vi "RunJustTailEllipseRatioRails.vi"() -> ()   [LabVIEW 2019]
uses:
  Parameters.ctl
  JustTailEllipseRatioRails/JustTailEllipseRatioRailsInputCluster.ctl
  JustTailEllipseRatioRails.lvclass
  D:/Github_repos/ProjectAPI/LabviewVIs/StimulusObject.lvclass
panel:
  in  "JustTailEllipseRatioRailsInputCluster":T1={"Constant Intensity (uW/mm^2, negative is blue)"=0.0, "dot radius (mm)"=0.2, "Intensities (uW/mm^2, negative is blue)"=[], "Durations (s)"=[], "Inter trigger interval (s)"=30.0, "Ellipse Ratio Trigger Point"=5.0}
  out "error IO":errorcluster
  in  "SSH password 2":string
  in  "SSH user name 2":string
  in  "Start":bool
  in  "Wait Before Recording (s)":u32
  in  "SSH password":string
  in  "SSH user name":string
  in  "Last Experiment of the Day":bool
  in  "Tags":string
  out "Parameters":T2 {"FW_WormLengthSD" format="%#.6e"}
  # "Faux Worm Drawing"
  # "Tracking"
  # "Temporal Calibration"
  # "Stimulus Generation"
  # "Median Filtering"
  # "Experimental Settings"
  # "Camera and Projector Settings"
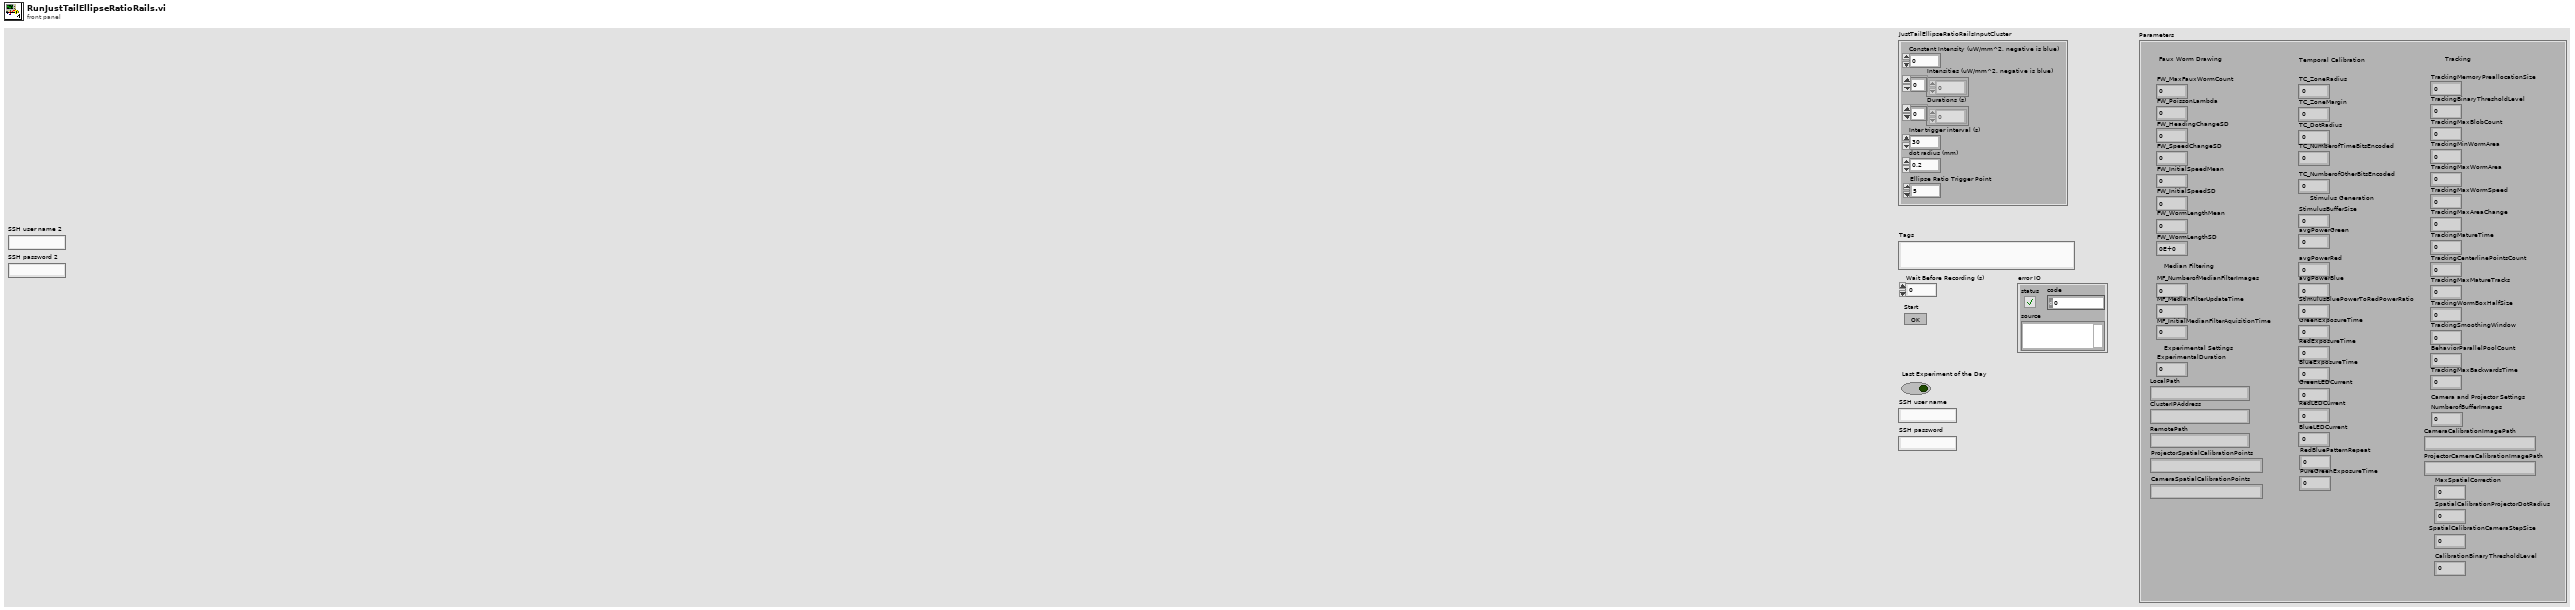
[diagram p1: front panel]
types:
  T1 = typedef "JustTailEllipseRatioRails.lvclass/JustTailEllipseRatioRailsInputCluster.ctl" = cluster{"Constant Intensity (uW/mm^2, negative is blue)":sgl, "dot radius (mm)":sgl, "Intensities (uW/mm^2, negative is blue)":sgl[], "Durations (s)":sgl[], "Inter trigger interval (s)":dbl, "Ellipse Ratio Trigger Point":sgl}
  T2 = typedef "Parameters.ctl" = cluster{"FW_MaxFauxWormCount":i32, "FW_PoissonLambda":dbl, "FW_HeadingChangeSD":dbl, "FW_SpeedChangeSD":dbl, "FW_InitialSpeedMean":dbl, "FW_InitialSpeedSD":dbl, "FW_WormLengthMean":dbl, "FW_WormLengthSD":dbl, "MF_NumberofMedianFilterImages":i32, "MF_MedianFilterUpdateTime":i32, "MF_InitialMedianFilterAquisitionTime":dbl, "ExperimentalDuration":i32, "TC_ZoneRadius":i32, "TC_ZoneMargin":i32, "TC_DotRadius":dbl, "TC_NumberofTimeBitsEncoded":i32, "TC_NumberofOtherBitsEncoded":i32, "NumberofBufferImages":sgl, "CameraCalibrationImagePath":string, "ProjectorCameraCalibrationImagePath":string, "StimulusBufferSize":i32, "TrackingMemoryPreallocationSize":i32, "TrackingBinaryThresholdLevel":sgl, "TrackingMaxBlobCount":i32, "TrackingMinWormArea":dbl, "TrackingMaxWormArea":dbl, "TrackingMaxWormSpeed":dbl, "TrackingMaxAreaChange":dbl, "TrackingMatureTime":i32, "TrackingCenterlinePointsCount":i32, "TrackingMaxMatureTracks":i32, "TrackingWormBoxHalfSize":i32, "TrackingSmoothingWindow":i32, "BehaviorParallelPoolCount":i32, "LocalPath":string, "GreenExposureTime":i32, "RedExposureTime":i32, "BlueExposureTime":i32, "ClusterIPAddress":string, "RemotePath":string, "GreenLEDCurrent":u8, "RedLEDCurrent":u8, "BlueLEDCurrent":u8, "avgPowerGreen":sgl, "avgPowerRed":sgl, "avgPowerBlue":sgl, "StimulusBluePowerToRedPowerRatio":sgl, "TrackingMaxBackwardsTime":i32, "MaxSpatialCorrection":dbl, "ProjectorSpatialCalibrationPoints":string, "SpatialCalibrationProjectorDotRadius":i32, "SpatialCalibrationCameraStepSize":dbl, "CameraSpatialCalibrationPoints":string, "CalibrationBinaryThresholdLevel":dbl, "RedBluePatternRepeat":i32, "PureGreenExposureTime":i32}
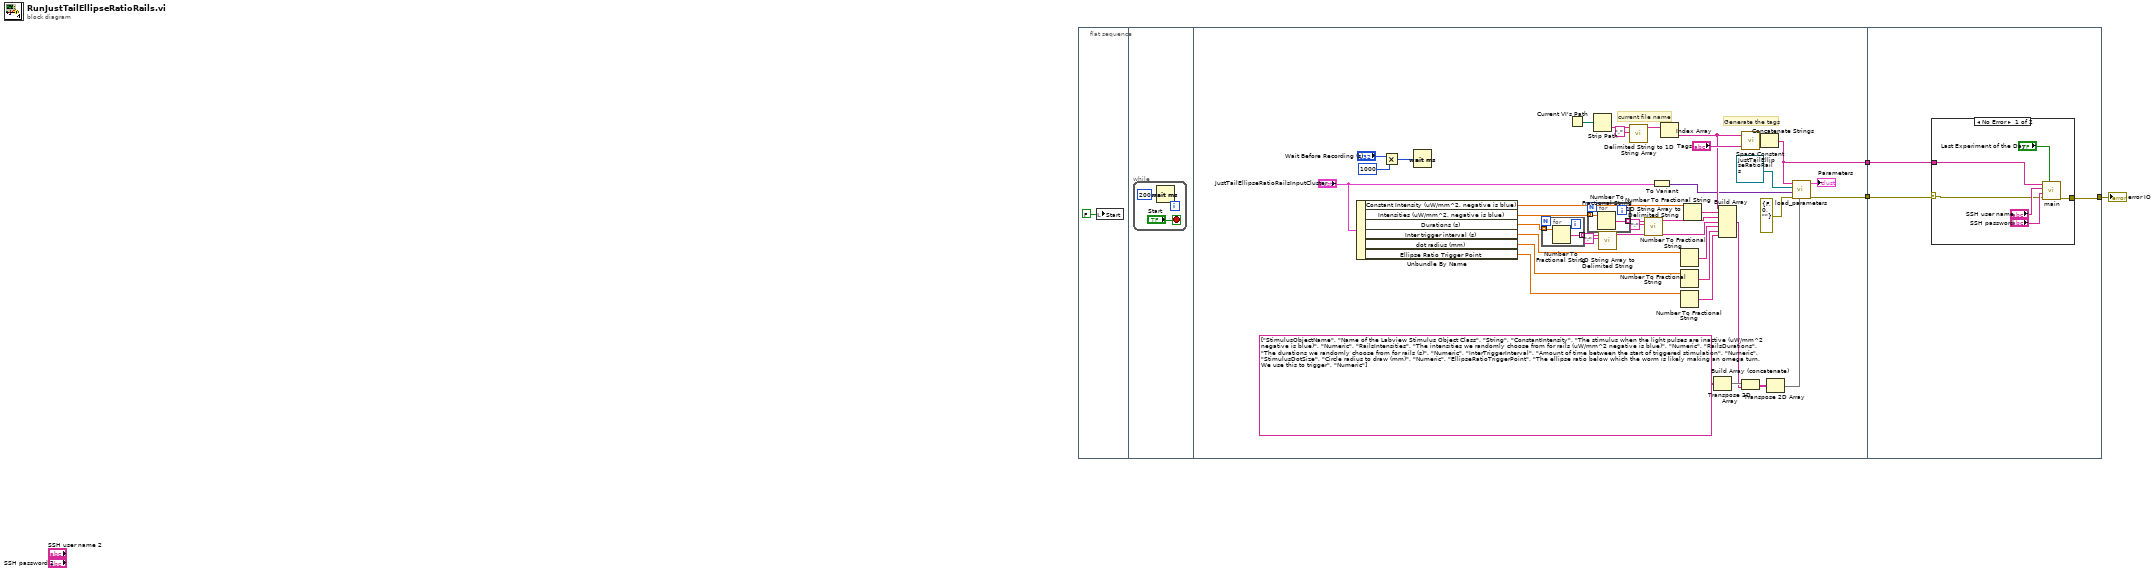
[diagram p0: block diagram]
diagram:
  n1 = flat-sequence {
    tunnel: [w44] -> w3
    tunnel: [w34] -> w2
    tunnel: w2 -> [w50]
    tunnel: w3 -> [w51]
    tunnel: [w49] -> w1
    frame #0 {
      n2 = local write "Start"(FALSE ("Start")) -> ()
    }
    frame #1 {
      n3 = while {
        stop <- "Start" stop-if-true
        n4 = Wait (ms)(milliseconds to wait=u32 200) -> ()  [unwired: 1 out]
      }
    }
    frame #2 {
      # "current file name"
      # "Generate the tags"
      n5 = Unbundle By Name("JustTailEllipseRatioRailsInputCluster") -> ("Constant Intensity (uW/mm^2, negative is blue)"=w23:sgl, "Intensities (uW/mm^2, negative is blue)"=w22:sgl[], "Durations (s)"=w16:sgl[], "Inter trigger interval (s)"=w13:dbl, "dot radius (mm)"=w14:sgl, "Ellipse Ratio Trigger Point"=w10:sgl)
      n6 = Multiply(x="Wait Before Recording (s)", y=u32 1000) -> (x*y=w31:u32)
      n7 = Wait (ms)(milliseconds to wait=w31) -> ()  [unwired: 1 out]
      n8 = for {
        tunnel: w16 -> [w46] mode=indexing
        tunnel: [w45] -> w18 mode=indexing
        n9 = Number To Fractional String(number=w46) -> (F-format string=w45:string)  [unwired: 3 in]
      }
      n10 = Current VI's Path() -> (path=w29:path)
      n11 = for {
        tunnel: w22 -> [w48] mode=indexing
        tunnel: [w47] -> w21 mode=indexing
        n12 = Number To Fractional String(number=w48) -> (F-format string=w47:string)  [unwired: 3 in]
      }
      n13 = Strip Path(path=w29) -> (name=w28:string)  [unwired: 1 out]
      n14 = call <vilib>:"1D String Array to Delimited String.vi"("delimiter"=";", "string array"=w18) -> ("delimited string"=w15:string)  [unwired: 9 in]
      n15 = call <vilib>:"Delimited String to 1D String Array.vi"("delimiter"=".", "delimited string"=w28) -> ("string array"=w26:string[])  [unwired: 9 in]
      n16 = call <vilib>:"1D String Array to Delimited String.vi"("delimiter"=";", "string array"=w21) -> ("delimited string"=w19:string)  [unwired: 9 in]
      n17 = To Variant(anything="JustTailEllipseRatioRailsInputCluster") -> (Variant=w24:variant)
      n18 = Index Array(array=w26) -> (element=w25:string)  [unwired: 1 in]
      n19 = Number To Fractional String(number=w13) -> (F-format string=w12:string)  [unwired: 3 in]
      n20 = Number To Fractional String(number=w14) -> (F-format string=w11:string)  [unwired: 3 in]
      n21 = Number To Fractional String(number=w10) -> (F-format string=w9:string)  [unwired: 3 in]
      n22 = Number To Fractional String(number=w23) -> (F-format string=w42:string)  [unwired: 3 in]
      n23 = Transpose 2D Array(2D array=string[][] [["StimulusObjectName", "Name of the Labview Stimulus Object Class", "String"], ["ConstantIntensity", "The stimulus when the light pulses are inactive (uW/mm^2 negative is blue)", "Numeric"], ["RailsIntensities", "The intensities we randomly choose from for rails (uW/mm^2 negative is blue)", "Numeric"], ["RailsDurations", "The durations we randomly choose from for rails (s)", "Numeric"], ["InterTriggerInterval", "Amount of time between the start of triggered stimulation", "Numeric"], ["StimulusDotSize", "Circle radius to draw (mm)", "Numeric"], ["EllipseRatioTriggerPoint", "The ellipse ratio below which the worm is likely making an omega turn. We use this to trigger", "Numeric"]]) -> (transposed array=w40:string[][])
      n24 = Build Array(w25, w42, w19, w15, w12, w11, w9) -> (w39:string[])
      n25 = Build Array (concatenate)(w40, w39) -> (w38:string[][])
      n26 = call <vilib>:"Space Constant.vi"() -> ("String"=w36:string)
      n27 = Concatenate Strings(w25, w36, "Tags") -> (w34:string)
      n28 = Transpose 2D Array(2D array=w38) -> (transposed array=w35:string[][])
      n29 = call "load_parameters.vi"("additional loaded parameters to write"=w35, "error in (no error)"=errorcluster {"status"=FALSE, "code"=0, "source"=""}, "StimulusObject Parameters"=w24, "StimulusObjectClassInput"=refnum<class "JustTailEllipseRatioRails.lvclass"> refnum ("JustTailEllipseRatioRails.lvclass"), "Tags"=w34) -> ("error out"=w44:errorcluster, "Parameters"=→"Parameters":T2)  [unwired: 4 in, 1 out]
    }
    frame #3 {
      n30 = case shown="No Error" w51 {
        selector: w51 -> [w54 w58]
        tunnel: [w53 w58] -> w49
        tunnel: w50 -> [w52 _]
        frame No Error {
          n31 = call "main.vi"("Last Experiment of the Day"="Last Experiment of the Day", "error in"=w54, "SSH password"="SSH password", "SSH user name"="SSH user name", "Tags"=w52) -> ("error out"=w53:errorcluster)  [unwired: 6 in]
        }
        frame Error {
        }
      }
    }
  }
  "error IO" <- w1
